vi "登陆界面.vi"() -> ()   [LabVIEW 2013]
panel:
  out "成功提示":bool
  in  "取消按钮":bool
  in  "确定按钮":bool
  in  "密码":string
  in  "用户名":string
  # "监控平台登陆界面"
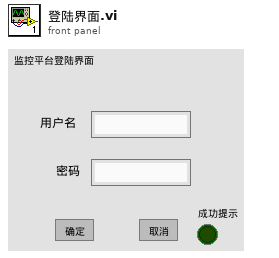
[diagram p1: front panel]
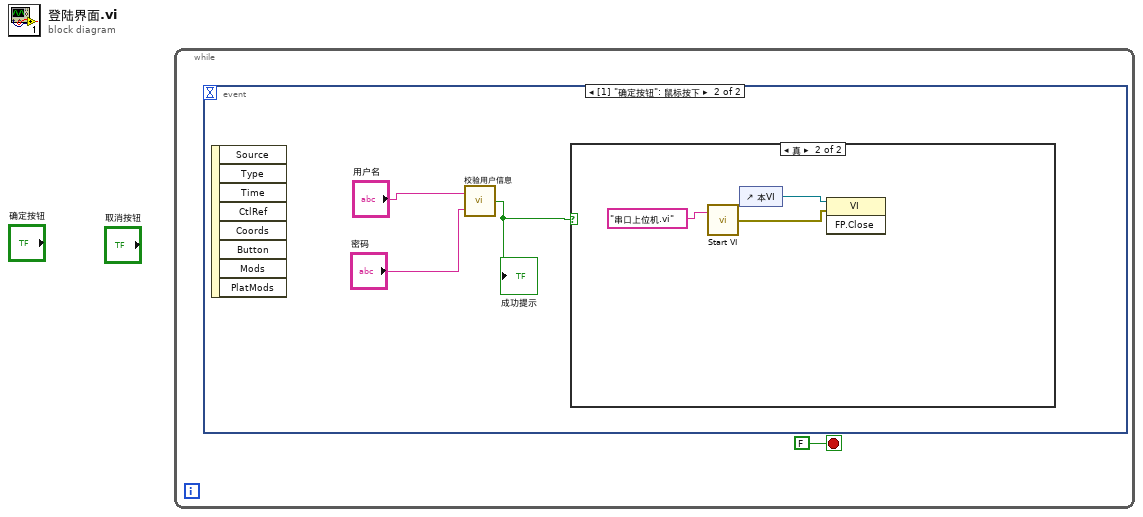
[diagram p0: block diagram]
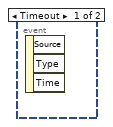
[diagram p2: hidden frame]
diagram:
  n1 = while {
    stop <- FALSE stop-if-true
    n2 = event shown="[1] \"确定按钮\": 鼠标按下" {
      selector: _ -> [_ _]
      dyn-events: _ -> [_ _]
      timeout: _ -> [_ _]
      event Timeout {
        n3 = event-data() -> ()  [unwired: 1 in, 3 out]
      }
      event "确定按钮": Mouse Down {
        n4 = event-data() -> ()  [unwired: 1 in, 8 out]
        n5 = call "校验用户信息.vi"("密码"="密码", "用户名"="用户名") -> ("布尔"=w2:bool)
        "成功提示" <- w2
        n6 = case shown="真" w2 {
          frame False {
          }
          frame True {
            n7 = call "Start VI.vi"("VI名称或相对路径"="串口上位机.vi") -> ("error out"=w5:errorcluster)  [unwired: 1 in]
            n8 = control-ref of="本VI"() -> (w7:refnum<vi>)
            n9 = invoke class="VI" method="FP.Close"(reference=w7, error in=w5) -> ()  [unwired: 1 in, 3 out]
          }
        }
      }
    }
  }
